vi "Unsubscribe from Context.vi"(8 "error in (no error)":errorcluster, 9 "Context":T1, 10 "Subscriber Enq":refnum<class "Message Enqueuer.lvclass">, 11 "Application Controller in":refnum<class "Application Controller.lvclass">) -> (0 "error out":errorcluster, 3 "Application Controller out":refnum<class "Application Controller.lvclass">)   [LabVIEW 2021, in "Application Controller.lvclass"]
uses:
  Publish-Subscribe/Context.ctl
  <vilib>/ActorFramework/Message Enqueuer/Message Enqueuer.lvclass
  Application Controller.lvclass
  Application Controller.lvclass/Application Controller.ctl
  Publish-Subscribe/Interfaces/Publisher Messages/Unsubscribe from Context Msg/Unsubscribe from Context Msg.lvclass
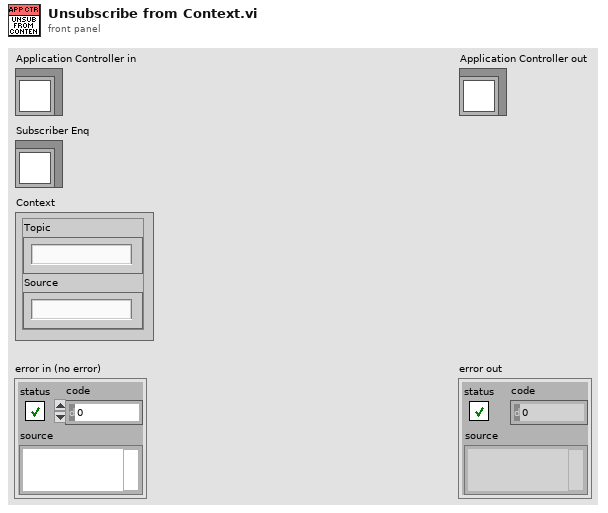
[diagram p1: front panel]
types:
  T1 = typedef "Context.ctl" = cluster{"Topic":string, "Source":string}
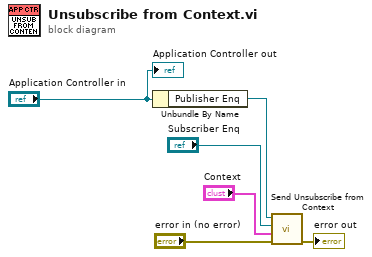
[diagram p0: block diagram]
diagram:
  n1 = Unbundle By Name("Application Controller in") -> ("Publisher Enq"=w5:refnum<class "Message Enqueuer.lvclass">)
  n2 = call "Send Unsubscribe from Context.vi"("error in (no error)"="error in (no error)", "Context"="Context", "Subscriber Enq"="Subscriber Enq", "Message Enqueuer"=w5) -> ("error out"=→"error out":errorcluster)  [unwired: 6 in, 1 out]
  "Application Controller out" <- "Application Controller in"
